vi "Phasor Compute tau_phi SDV.vi"(8 "Error In":errorcluster, 9 "Phasor Frequency":dbl[unit], 10 "Phasor SDV (g, s)":T1, 11 "Phasor (g, s)":T1) -> (0 "Error Out":errorcluster, 3 "tau_phi SDV":dbl[unit])   [LabVIEW 2021, in "Phasor.lvlib"]
uses:
  Phasor (g, s).ctl
  Phasor.lvlib
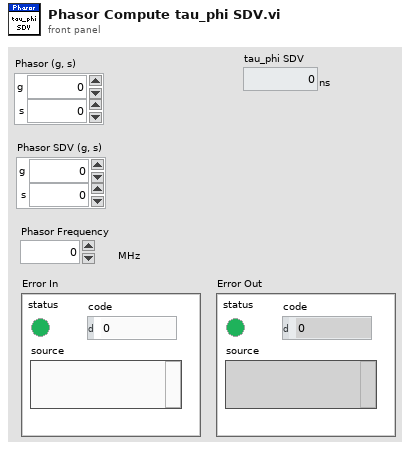
[diagram p1: front panel]
types:
  T1 = typedef "Phasor.lvlib/Phasor (g, s).ctl" = cluster{"g":dbl, "s":dbl}
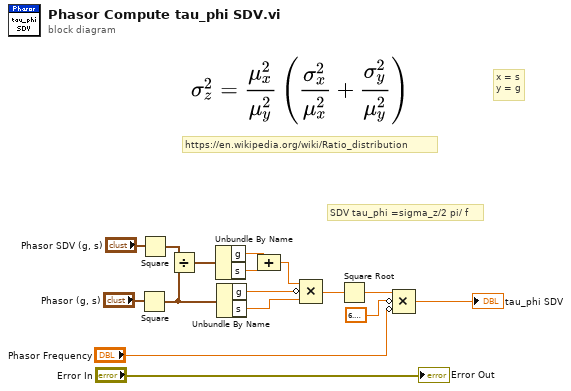
[diagram p0: block diagram]
diagram:
  # "SDV tau_phi =sigma_z/2 pi/ f"
  # "x = s\ny = g"
  # "https://en.wikipedia.org/wiki/Ratio_distribution"
  n1 = Square(x="Phasor (g, s)") -> (x^2=w11:T1)
  n2 = Square(x="Phasor SDV (g, s)") -> (x^2=w13:T1)
  n3 = Divide(x=w13, y=w11) -> (x/y=w12:T1)
  n4 = Unbundle By Name(w12) -> ("g"=w8:dbl, "s"=w7:dbl)
  n5 = Unbundle By Name(w11) -> ("g"=w10:dbl, "s"=w9:dbl)
  n6 = Compound Arithmetic op=ADD(w8, w7) -> (w6:dbl)
  n7 = Compound Arithmetic op=MULTIPLY(w6, invert w10, w9) -> (w5:dbl)
  n8 = Square Root(x=w5) -> (sqrt(x)=w4:dbl)
  n9 = Compound Arithmetic op=MULTIPLY(w4, invert 6.283185307179586, invert "Phasor Frequency") -> (→"tau_phi SDV":dbl[unit])
  "Error Out" <- "Error In"
